vi "CloseConnection.vi"(8 "error in (no error)":errorcluster, 11 "STOMP in":refnum<class "STOMP.lvclass">) -> (0 "error out":errorcluster, 3 "STOMP out":refnum<class "STOMP.lvclass">)   [LabVIEW 2017, in "STOMP.lvclass"]
uses:
  STOMP.lvclass
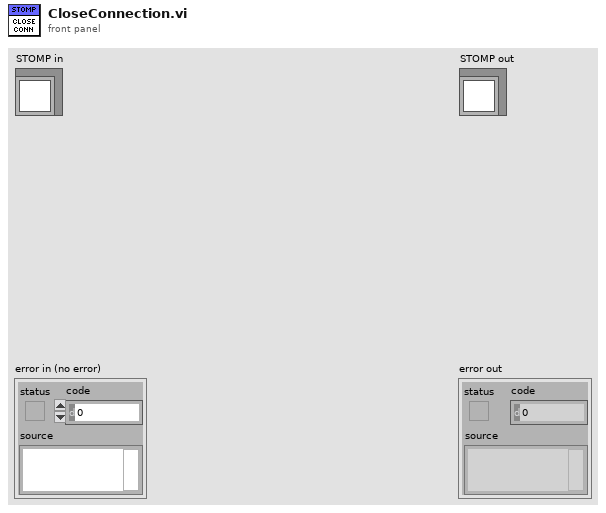
[diagram p1: front panel]
types:
  T1 = typedef "STOMP.lvclass/ObjectAttributes.ctl" = cluster{"address":string, "port":u16, "ConnectionRef":refnum<k5>, "messageQueue":refnum<queue>, "receiptQueue":refnum<queue>, "errorQueue":refnum<queue>, "sendQueue":refnum<queue>, "currentReceiptNumber":u64, "currentSubscriptionId":u64, "closeConnection":bool, "activeSubscriptions":T2[]}
  T2 = typedef "STOMP.lvclass/Type_ActiveSubscription.ctl" = cluster{"id":u64, "receipt":bool, "Destination":string, "ack":T3, "headers":T4[]}
  T3 = typedef "STOMP.lvclass/Type_AckHeader.ctl" = enum16{"auto", "client", "client-individual"}
  T4 = typedef "STOMP.lvclass/Type_FrameHeader.ctl" = cluster{"Header":string, "Value":string}
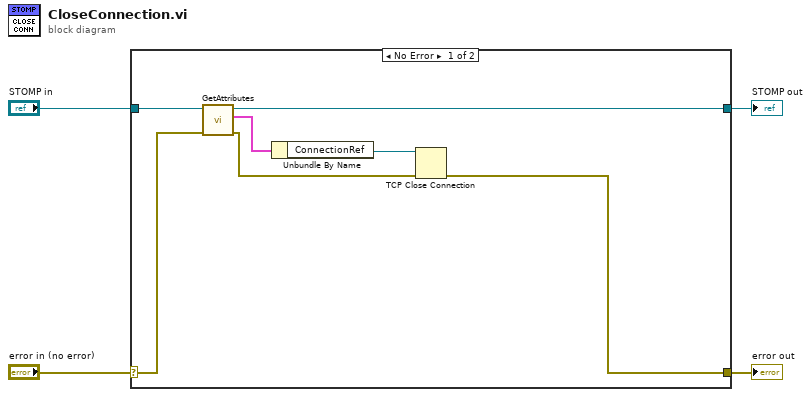
[diagram p0: block diagram]
diagram:
  n1 = case shown="No Error" "error in (no error)" {
    selector: "error in (no error)" -> [w6 w13]
    tunnel: [w10 w13] -> w3
    tunnel: [w7 w12] -> w1
    tunnel: "STOMP in" -> [w9 w12]
    frame No Error {
      n2 = call-dynamic "GetAttributes.vi"("error in (no error)"=w6, "STOMP in"=w9) -> ("error out"=w5:errorcluster, "attributes"=w8:T1, "STOMP out"=w7:refnum<class "STOMP.lvclass">)  [unwired: 7 in]
      n3 = Unbundle By Name(w8) -> ("ConnectionRef"=w11:refnum<k5>)
      n4 = TCP Close Connection(connection ID=w11, error in (no error)=w5) -> (error out=w10:errorcluster)  [unwired: 1 in, 1 out]
    }
    frame Error {
    }
  }
  "error out" <- w3
  "STOMP out" <- w1
